vi "Exercice2.vi"() -> ()   [LabVIEW 2018]
panel:
  out "led":bool
  in  "c":dbl(knob) min=0.0 max=9.0 step=1.0 scale=0.0..10.0
  in  "b":dbl(knob) min=0.0 max=9.0 step=1.0 scale=0.0..10.0
  in  "a":dbl(knob) min=0.0 max=9.0 step=1.0 scale=0.0..10.0
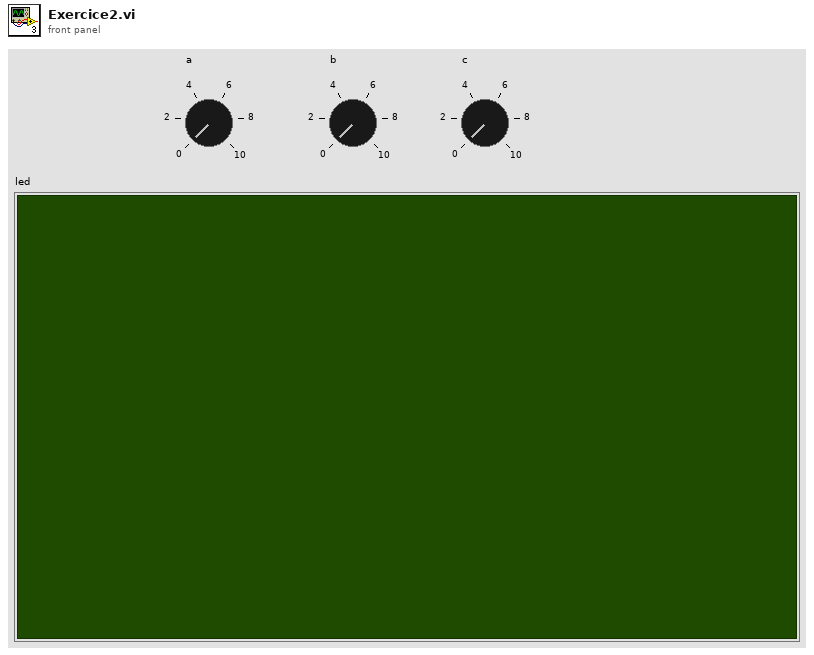
[diagram p1: front panel]
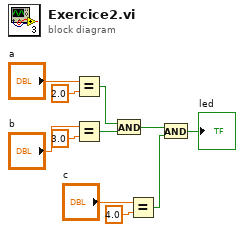
[diagram p0: block diagram]
diagram:
  n1 = Equal?(x="a", y=2.0) -> (x = y?=w5:bool)
  n2 = Equal?(x="b", y=3.0) -> (x = y?=w4:bool)
  n3 = And(x=w5, y=w4) -> (x .and. y?=w2:bool)
  n4 = Equal?(x="c", y=4.0) -> (x = y?=w3:bool)
  n5 = And(x=w2, y=w3) -> (x .and. y?=→"led":bool)
